vi "sir_v7.vi"() -> ()   [LabVIEW 2009]
panel:
  in  "Pozitia":dbl=16.0
  in  "Numarul de caractere":dbl=26.0
  in  "stop":bool
  out "Sirul  extras":string="subsir din cadrul unui sir"
  in  "Sirul initial":string="Extragerea unui subsir din cadrul unui sir de caractere"
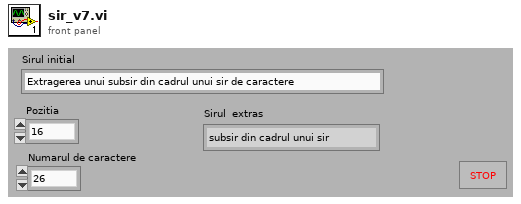
[diagram p1: front panel]
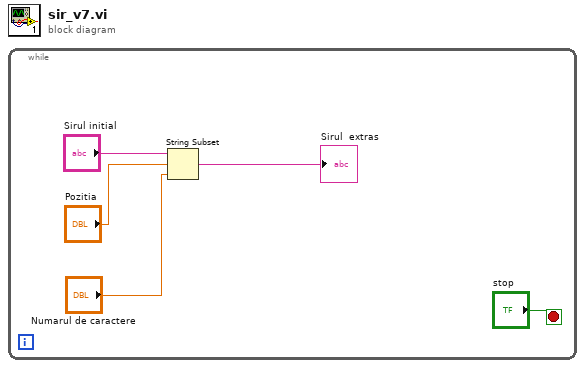
[diagram p0: block diagram]
diagram:
  n1 = while {
    stop <- "stop" stop-if-true
    n2 = String Subset(string="Sirul initial", offset (0)="Pozitia", length (rest)="Numarul de caractere") -> (substring=→"Sirul  extras":string)
  }
